vi "Judge_Step.vi"(9 "Asymmetry":dbl, 11 "Position":dbl) -> (0 "Off To On?":bool, 3 "New Position":dbl)   [LabVIEW 2020]
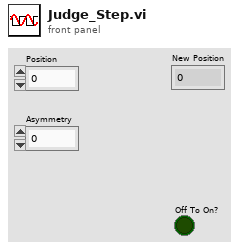
[diagram p1: front panel]
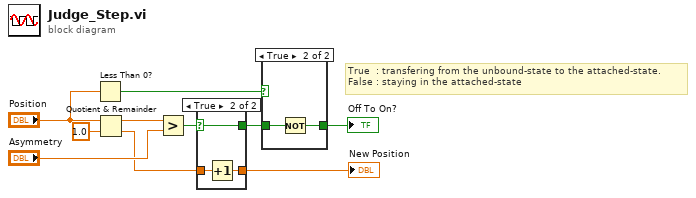
[diagram p0: block diagram]
diagram:
  # "True  : transfering from the unbound-state to the attached-state.\nFalse : staying in the attached-state"
  n1 = Less Than 0?(x="Position") -> (x < 0?=w5:bool)
  n2 = Quotient & Remainder(x="Position", y=1.0) -> (x-y*floor(x/y)=w7:dbl, floor(x/y)=w2:dbl)
  n3 = Greater?(x=w7, y="Asymmetry") -> (0:w8:bool)
  n4 = case shown="TRUE" w8 {
    selector: w8 -> [w11 w13]
    tunnel: w2 -> [w12 w15]
    tunnel: [w12 w14] -> w1
    tunnel: [w11 w13] -> w4
    frame False {
    }
    frame True {
      n5 = Increment(x=w15) -> (x+1=w14:dbl)
    }
  }
  "New Position" <- w1
  n6 = case shown="TRUE" w5 {
    tunnel: w4 -> [w16 w18]
    tunnel: [w16 w17] -> w3
    frame False {
    }
    frame True {
      n7 = Not(x=w18) -> (.not. x?=w17:bool)
    }
  }
  "Off To On?" <- w3
